vi "Load Instruments.vi"(8 "error in (no error)":errorcluster, 11 "ManualUI in":refnum<class "ManualUI.lvclass">) -> (0 "error out":errorcluster, 3 "ManualUI out":refnum<class "ManualUI.lvclass">)   [LabVIEW 2023, in "ManualUI.lvlib" / "ManualUI.lvclass"]
uses:
  Library/ManualUI.lvclass
  Library/ManualUI.lvclass/ManualUI.ctl
  builds/Framework/Configuration.lvlibp/Library/Configuration.lvclass
  builds/Framework/Engine.lvlibp/Engine/Library/Engine.lvclass
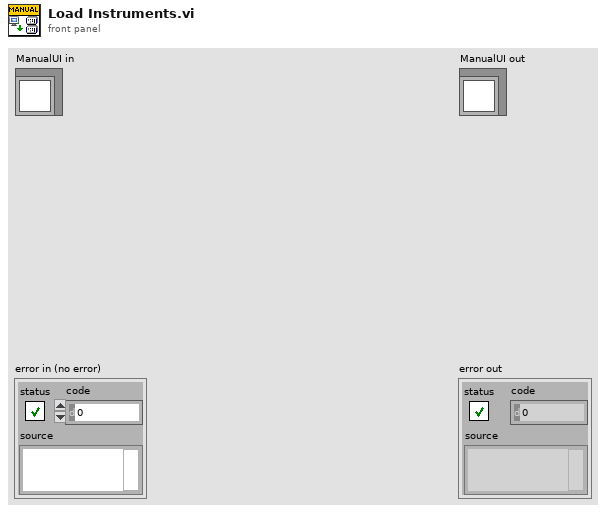
[diagram p1: front panel]
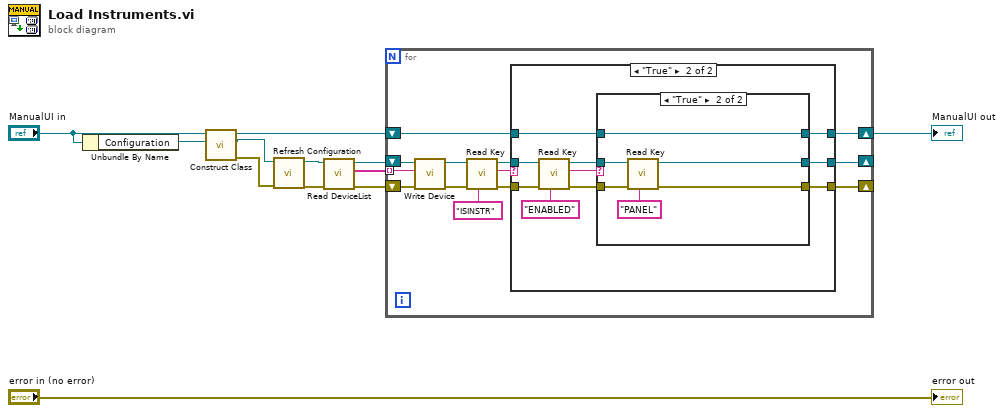
[diagram p0: block diagram]
diagram:
  n1 = Unbundle By Name("ManualUI in") -> ("Configuration"=w11:refnum<class "Configuration.lvclass">)
  n2 = call "Construct Class.vi"("Actor in"=w11, "Engine in"="ManualUI in") -> ("error out"=w9:errorcluster, "Actor out"=w10:refnum<class "Configuration.lvclass">, "Engine out"=w8:refnum<class "ManualUI.lvclass">)  [unwired: 7 in]
  n3 = call "Refresh Configuration.vi"("error in (no error)"=w9, "Configuration in"=w10) -> ("error out"=w4:errorcluster, "Configuration out"=w5:refnum<class "Configuration.lvclass">)  [unwired: 8 in]
  n4 = call "Read DeviceList.vi"("error in (no error)"=w4, "Configuration in"=w5) -> ("error out"=w3:errorcluster, "DeviceList"=w1:string[], "Configuration out"=w2:refnum<class "Configuration.lvclass">)  [unwired: 7 in]
  n5 = for {
    shift-right: [w19] -> _
    shift-left: w2 -> [w25]
    shift-right: [w17] -> _
    shift-left: w3 -> [w16]
    shift-right: [w14] -> w7
    shift-left: w8 -> [w15]
    tunnel: w1 -> [w13] mode=indexing
    n6 = call "Write Device.vi"("error in (no error)"=w16, "Device"=w13, "Configuration in"=w25) -> ("error out"=w23:errorcluster, "Configuration out"=w24:refnum<class "Configuration.lvclass">)  [unwired: 7 in]
    n7 = call "Read Key.vi"("Key"="ISINSTR", "error in (no error)"=w23, "Configuration in"=w24) -> ("error out"=w18:errorcluster, "Value"=w21:string, "Configuration out"=w20:refnum<class "Configuration.lvclass">)  [unwired: 6 in]
    n8 = case shown="\"True\"" w21 {
      tunnel: w20 -> [w28 w36]
      tunnel: [w28 w33] -> w19
      tunnel: w18 -> [w27 w37]
      tunnel: [w27 w31] -> w17
      tunnel: w15 -> [w26 w30]
      tunnel: [w26 w29] -> w14
      frame "False", Default {
      }
      frame "True" {
        n9 = call "Read Key.vi"("Key"="ENABLED", "error in (no error)"=w37, "Configuration in"=w36) -> ("error out"=w32:errorcluster, "Value"=w35:string, "Configuration out"=w34:refnum<class "Configuration.lvclass">)  [unwired: 6 in]
        n10 = case shown="\"True\"" w35 {
          tunnel: w34 -> [w41 w45]
          tunnel: [w41 w44] -> w33
          tunnel: w32 -> [w40 w46]
          tunnel: [w40 w43] -> w31
          tunnel: w30 -> [w39 w42]
          tunnel: [w39 w42] -> w29
          frame "False", Default {
          }
          frame "True" {
            n11 = call "Read Key.vi"("Key"="PANEL", "error in (no error)"=w46, "Configuration in"=w45) -> ("error out"=w43:errorcluster, "Configuration out"=w44:refnum<class "Configuration.lvclass">)  [unwired: 6 in, 1 out]
          }
        }
      }
    }
  }
  "ManualUI out" <- w7
  "error out" <- "error in (no error)"
